vi "Init Output Poller.vi"(8 "error in (no error)":errorcluster, 11 "output_actor in":refnum<class "Output Actor.lvclass">) -> (0 "error out":errorcluster, 3 "output_actor out":refnum<class "Output Actor.lvclass">)   [LabVIEW 2015, in "Output Actor.lvclass"]
uses:
  Output Actor.lvclass
  <vilib>/ActorFramework/Actor/Actor.lvclass/Actor.ctl
  <vilib>/ActorFramework/Message Enqueuer/Message Enqueuer.lvclass/Message Enqueuer.ctl
  Output Actor.lvclass/Output Actor.ctl
  output/output_poller/output_poller_actor/output_poller_actor.lvclass
  output/output_poller/output_poller_actor/output_poller_actor.lvclass/output_poller_actor.ctl
  <vilib>/ActorFramework/Message Enqueuer/Init from Existing Queue.vi
  <vilib>/ActorFramework/Message Enqueuer/Message Enqueuer.lvclass
  <vilib>/ActorFramework/Actor/Actor.lvclass
  output/Output.lvclass
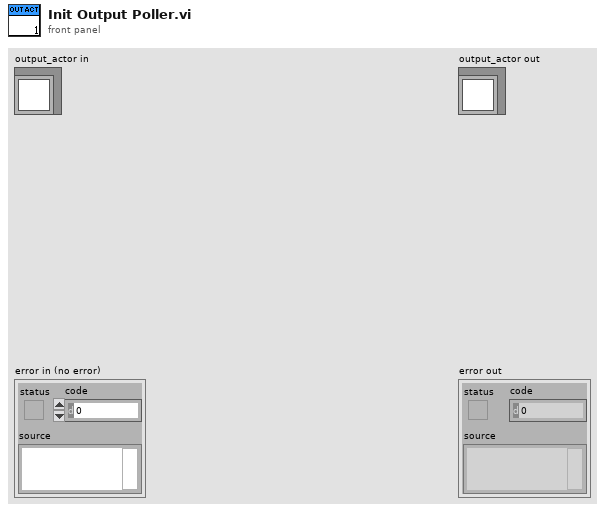
[diagram p1: front panel]
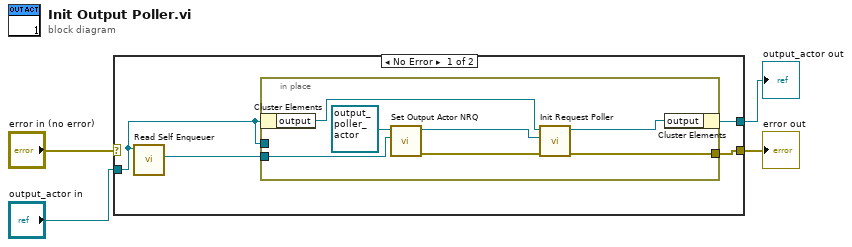
[diagram p0: block diagram]
diagram:
  n1 = case shown="No Error" "error in (no error)" {
    selector: "error in (no error)" -> [_ w17]
    tunnel: [w6 w17] -> w3
    tunnel: [w5 w16] -> w1
    tunnel: "output_actor in" -> [w7 w16]
    frame No Error {
      n2 = call <vilib>:"Read Self Enqueuer.vi"("Actor"=w7) -> ("Self Enqueuer"=w8:refnum<class "Message Enqueuer.lvclass">)  [unwired: 10 in]
      n3 = in-place {
        in-place-border: w7 -> [_]
        in-place-border: w8 -> [w14]
        in-place-border: [w9] -> w6
        n4 = in-place-cluster #1(w7) -> ("output"=w11:refnum<class "Output.lvclass">)
        n5 = call "Set Output Actor NRQ.vi"("Actor Framework:Message Enqueuer"=w14, "output_poller_actor in"=refnum<class "output_poller_actor.lvclass"> refnum) -> ("error out"=w13:errorcluster, "output_poller_actor out"=w12:refnum<class "output_poller_actor.lvclass">)  [unwired: 8 in]
        n6 = call "Init Request Poller.vi"("error in (no error)"=w13, "output_request_poller in"=w12, "output in"=w11) -> ("error out"=w9:errorcluster, "output out"=w10:refnum<class "Output.lvclass">)  [unwired: 7 in]
        n7 = in-place-cluster #1("output"=w10) -> (w5:refnum<class "Output Actor.lvclass">)
      }
    }
    frame Error {
    }
  }
  "error out" <- w3
  "output_actor out" <- w1
